vi "AttrMap-ImportCluster.vi"(8 "error in (no error)":errorcluster, 10 "Cluster":variant, 11 "AttrMap in":T1) -> (0 "error out":errorcluster, 3 "AttrMap out":T1)   [LabVIEW 2019]
uses:
  Typedef/Def-AttrMap.ctl
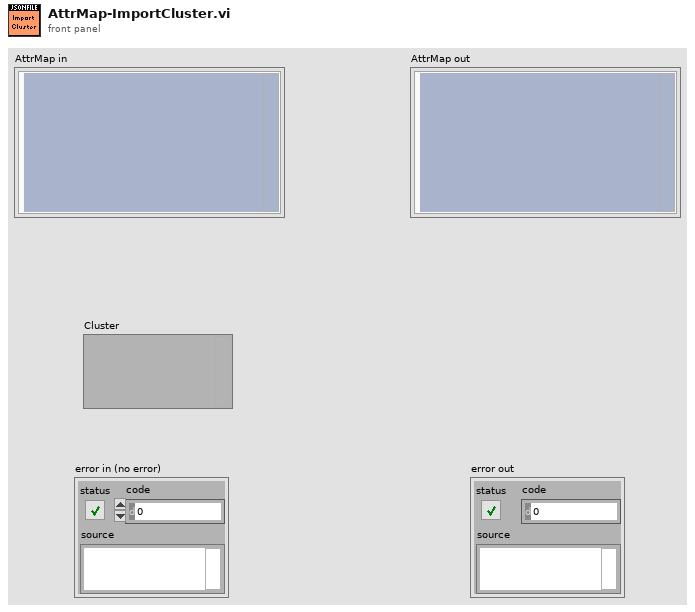
[diagram p1: front panel]
types:
  T1 = typedef "Def-AttrMap.ctl" = cluster{"Map":variant}
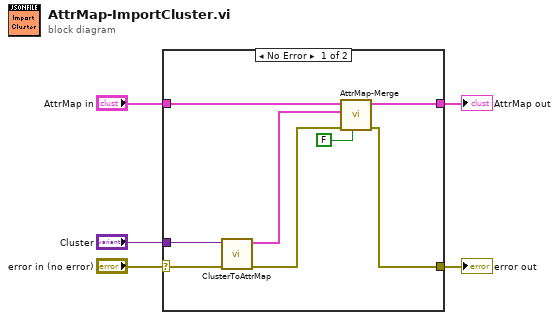
[diagram p0: block diagram]
diagram:
  n1 = case shown="No Error" "error in (no error)" {
    selector: "error in (no error)" -> [w12 w14]
    tunnel: [w7 w14] -> w5
    tunnel: "Cluster" -> [w13 _]
    tunnel: "AttrMap in" -> [w11 w15]
    tunnel: [w6 w15] -> w1
    frame No Error {
      n2 = call "ClusterToAttrMap.vi"("error in (no error)"=w12, "data"=w13) -> ("error out"=w8:errorcluster, "AttrMap"=w10:T1)  [unwired: 8 in]
      n3 = call "AttrMap-Merge.vi"("If exist? Skip(T)/Overwrite(F)"=FALSE, "error in (no error)"=w8, "AttrMap B"=w10, "AttrMap A"=w11) -> ("error out"=w7:errorcluster, "AttrMap A after B->A"=w6:T1)  [unwired: 6 in]
    }
    frame Error {
    }
  }
  "error out" <- w5
  "AttrMap out" <- w1
